vi "RPC Method Template.vi"(8 "error in (no error)":errorcluster, 10 "Request Data":cluster{"Numeric":dbl}, 11 "gRPC Client in":refnum<class "Template Client.lvclass">) -> (0 "error out":errorcluster, 2 "Response Data":cluster{"Numeric":dbl}, 3 "gRPC Client out":refnum<class "Template Client.lvclass">)   [LabVIEW 2019, in "Template Client.lvlib" / "Template Client.lvclass"]
uses:
  Template Client.lvclass
  Template Client.lvclass/Template Client.ctl
  fa22ca14-33b2-4bc3-8699-3f27c9b27c9c.vi
  gRPC lvSupport/Server API/Server/Get Server DLL Path.vi
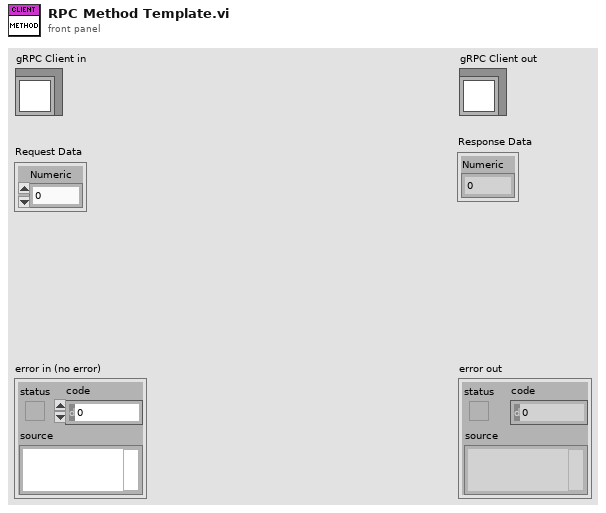
[diagram p1: front panel]
types:
  T1 = typedef "Template Client.lvlib/gprc-lvsupport.lvlib/grpcId.ctl" = u64
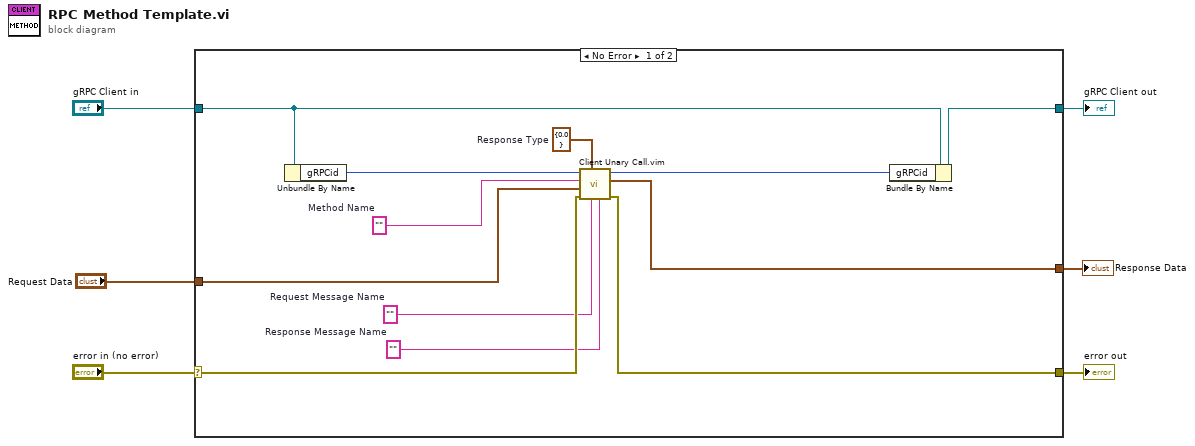
[diagram p0: block diagram]
diagram:
  n1 = case shown="No Error" "error in (no error)" {
    selector: "error in (no error)" -> [w14 w20]
    tunnel: [w13 w20] -> w5
    tunnel: [w15 w19] -> w3
    tunnel: "gRPC Client in" -> [w17 w19]
    tunnel: "Request Data" -> [w11 _]
    tunnel: [w10 _] -> w1
    frame No Error {
      w7 = ""  # Response Message Name
      w8 = ""  # Request Message Name
      w9 = cluster{"Numeric":dbl} {"Numeric"=0.0}  # Response Type
      w12 = ""  # Method Name
      n2 = Unbundle By Name(w17) -> ("gRPCid"=w18:T1)
      n3 = call "Client Unary Call.vim"("Response Message Name"=w7, "Request Message Name"=w8, "Response Type"=w9, "error in (no error)"=w14, "Request Data"=w11, "Method Name"=w12, "Client Ref"=w18) -> ("error out"=w13:errorcluster, "Response Data"=w10:cluster{"Numeric":dbl}, "Client Ref Out"=w16:u64)  [unwired: 2 in]
      n4 = Bundle By Name(cluster=w17, "gRPCid"=w16) -> (w15:refnum<class "Template Client.lvclass">)
    }
    frame Error {
    }
  }
  "error out" <- w5
  "gRPC Client out" <- w3
  "Response Data" <- w1
